vi "Right Initialization (SubVI).vi"   [LabVIEW 2015]
uses:
  Right Variables.vi
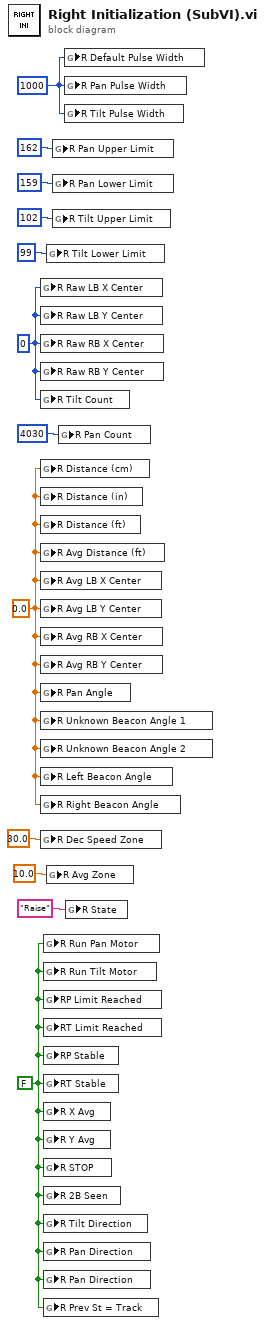
[diagram p0: block diagram]
diagram:
  w2 = u32 1000 ("Pan Upper Limit")
  w11 = u16 0 ("L Raw LB X Center")
  w1 = FALSE ("L Limit Reached")
  w6 = 0.0 ("R Distance (cm)")
  n1 = global write "Right Variables.vi" "R Raw LB X Center"(w11) -> ()
  n2 = global write "Right Variables.vi" "R Raw LB Y Center"(w11) -> ()
  n3 = global write "Right Variables.vi" "R Raw RB X Center"(w11) -> ()
  n4 = global write "Right Variables.vi" "R Raw RB Y Center"(w11) -> ()
  n5 = global write "Right Variables.vi" "R Tilt Count"(w11) -> ()
  n6 = global write "Right Variables.vi" "R Distance (cm)"(w6) -> ()
  n7 = global write "Right Variables.vi" "R Distance (in)"(w6) -> ()
  n8 = global write "Right Variables.vi" "R Distance (ft)"(w6) -> ()
  n9 = global write "Right Variables.vi" "R Avg Distance (ft)"(w6) -> ()
  n10 = global write "Right Variables.vi" "R Avg LB X Center"(w6) -> ()
  n11 = global write "Right Variables.vi" "R Avg LB Y Center"(w6) -> ()
  n12 = global write "Right Variables.vi" "R Avg RB X Center"(w6) -> ()
  n13 = global write "Right Variables.vi" "R Avg RB Y Center"(w6) -> ()
  n14 = global write "Right Variables.vi" "R Pan Angle"(w6) -> ()
  n15 = global write "Right Variables.vi" "R Unknown Beacon Angle 1"(w6) -> ()
  n16 = global write "Right Variables.vi" "R Unknown Beacon Angle 2"(w6) -> ()
  n17 = global write "Right Variables.vi" "R Left Beacon Angle"(w6) -> ()
  n18 = global write "Right Variables.vi" "R Right Beacon Angle"(w6) -> ()
  n19 = global write "Right Variables.vi" "R Dec Speed Zone"(30.0 ("Dead Zone")) -> ()
  n20 = global write "Right Variables.vi" "R Run Pan Motor"(w1) -> ()
  n21 = global write "Right Variables.vi" "R Run Tilt Motor"(w1) -> ()
  n22 = global write "Right Variables.vi" "RP Limit Reached"(w1) -> ()
  n23 = global write "Right Variables.vi" "RT Limit Reached"(w1) -> ()
  n24 = global write "Right Variables.vi" "RP Stable"(w1) -> ()
  n25 = global write "Right Variables.vi" "RT Stable"(w1) -> ()
  n26 = global write "Right Variables.vi" "R X Avg"(w1) -> ()
  n27 = global write "Right Variables.vi" "R Y Avg"(w1) -> ()
  n28 = global write "Right Variables.vi" "R STOP"(w1) -> ()
  n29 = global write "Right Variables.vi" "R 2B Seen"(w1) -> ()
  n30 = global write "Right Variables.vi" "R Tilt Direction"(w1) -> ()
  n31 = global write "Right Variables.vi" "R Pan Direction"(w1) -> ()
  n32 = global write "Right Variables.vi" "R Pan Direction"(w1) -> ()
  n33 = global write "Right Variables.vi" "R Prev St = Track"(w1) -> ()
  n34 = global write "Right Variables.vi" "R Tilt Lower Limit"(u16 99 ("Tilt Lower Limit")) -> ()
  n35 = global write "Right Variables.vi" "R Avg Zone"(10.0 ("Dead Zone")) -> ()
  n36 = global write "Right Variables.vi" "R Pan Upper Limit"(u16 162 ("Pan Upper Limit")) -> ()
  n37 = global write "Right Variables.vi" "R Pan Lower Limit"(u16 159 ("Pan Lower Limit")) -> ()
  n38 = global write "Right Variables.vi" "R Tilt Upper Limit"(u16 102 ("Tilt Upper Limit")) -> ()
  n39 = global write "Right Variables.vi" "R Pan Count"(4030 ("L Pan Count")) -> ()
  n40 = global write "Right Variables.vi" "R Default Pulse Width"(w2) -> ()
  n41 = global write "Right Variables.vi" "R Pan Pulse Width"(w2) -> ()
  n42 = global write "Right Variables.vi" "R Tilt Pulse Width"(w2) -> ()
  n43 = global write "Right Variables.vi" "R State"("Raise" ("R State")) -> ()
